vi "Main_Backup01.vi"() -> ()   [LabVIEW 2024]
uses:
  PIMax3Test01/x64/Debug/PIMax3Test02.dll
panel:
  out "Intensity Graph 2":u16[][](graph)
  out "image":u16[](array[numeric])
  out "Uninit Message":string
  out "close":string
  out "model":string
  out "open":string
  out "Init Message":string
  out "Uninit Code":i32
  out "Init Code":i32
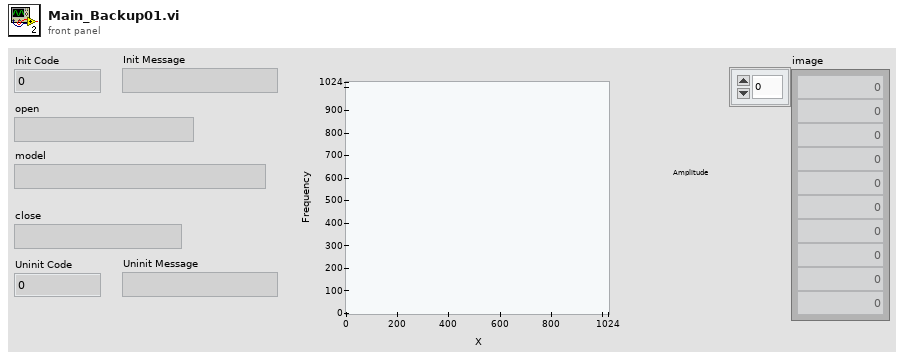
[diagram p1: front panel]
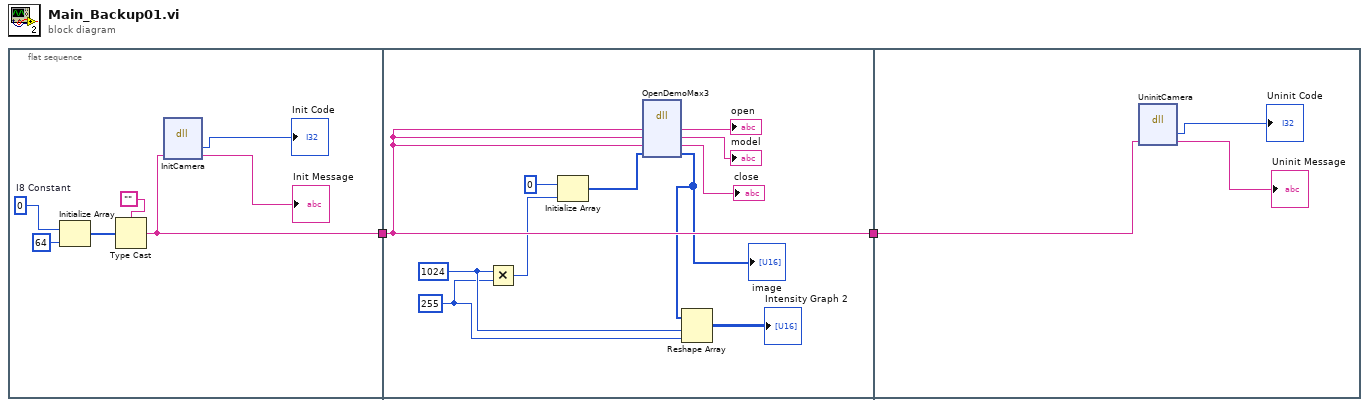
[diagram p0: block diagram]
diagram:
  n1 = flat-sequence {
    tunnel: [w3] -> w2
    tunnel: w2 -> [w17]
    tunnel: [w17] -> w1
    tunnel: w1 -> [w22]
    frame #0 {
      w8 = i8 0  # I8 Constant
      n2 = Initialize Array(w8, 64 ("dimension size")) -> (w7:i8[])
      n3 = Type Cast(type="", x=w7) -> (*(type *) &x=w3:string)
      n4 = dll-call lib="C:/Users/amir0/source/repos/PIMax3Test01/x64/Debug/PIMax3Test02.dll" fn="InitCamera"("Init Message"=w3) -> ("Init Code"=→"Init Code":i32, "Init Message"=→"Init Message":string)  [unwired: 5 in, 2 out]
    }
    frame #1 {
      w10 = 255
      w11 = 1024
      n5 = Multiply(x=w11, y=w10) -> (x*y=w12:i32)
      n6 = Initialize Array(u16 0, w12) -> (w15:u16[])
      n7 = dll-call lib="C:/Users/amir0/source/repos/PIMax3Test01/x64/Debug/PIMax3Test02.dll" fn="OpenDemoMax3"("open"=w17, "model"=w17, "close"=w17, "image"=w15) -> ("open"=→"open":string, "model"=→"model":string, "close"=→"close":string, "image"=w14:u16[])  [unwired: 4 in, 2 out]
      "image" <- w14
      n8 = Reshape Array(w14, w11, w10) -> (→"Intensity Graph 2":u16[][])
    }
    frame #2 {
      n9 = dll-call lib="C:/Users/amir0/source/repos/PIMax3Test01/x64/Debug/PIMax3Test02.dll" fn="UninitCamera"("Uninit Message"=w22) -> ("Uninit Code"=→"Uninit Code":i32, "Uninit Message"=→"Uninit Message":string)  [unwired: 5 in, 2 out]
    }
  }
